vi "current (SubVI).vi"(5 "T_wave":dbl=5.0, 6 "eta in":dbl[](array[numeric]), 7 "zeta_a":dbl, 8 "nu_c_ned in":dbl[](array[numeric])=[0.0, 0.0, 0.0, 0.0, 0.0, 0.0], 9 "dt sim":dbl=10.0, 10 "loop it":i32, 11 "Waves":bool) -> (3 "nu_c_ned out":dbl[](array[numeric]))   [LabVIEW 2014]
uses:
  <vilib>/imath/engines/lvmath2/RunTimeEngine/IndexRead/NIMS V(S).vi
  <instcachedir>/0/NIMS V(S)_0488751826AF41519A22953C041130DC.lvgen/NIMS V(S)_0488751826AF41519A22953C041130DC_000.vi
  <vilib>/imathl/engines/lvmath/Functions/Error Handling/Create Error.vi
  <vilib>/imath/engines/lvmath2/RunTimeEngine/NodeEndStatement/NIMS_NodeEndStatement_Output.vi
  <instcachedir>/0/NIMS_NodeEndStatement_Output_53EC0D466D134D7ABD903AC30B43404B.lvgen/NIMS_NodeEndStatement_Output_53EC0D466D134D7ABD903AC30B43404B_005.vi
  <vilib>/imath/engines/lvmath2/RunTimeEngine/ErrorHandling/NIMS_Finalize Error.vi
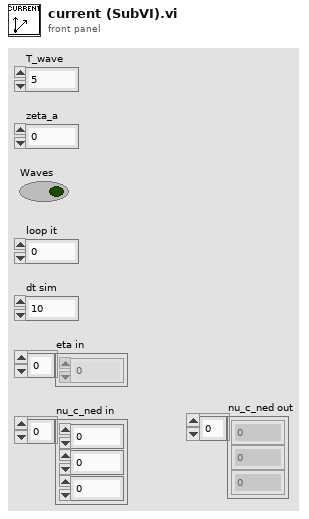
[diagram p1: front panel]
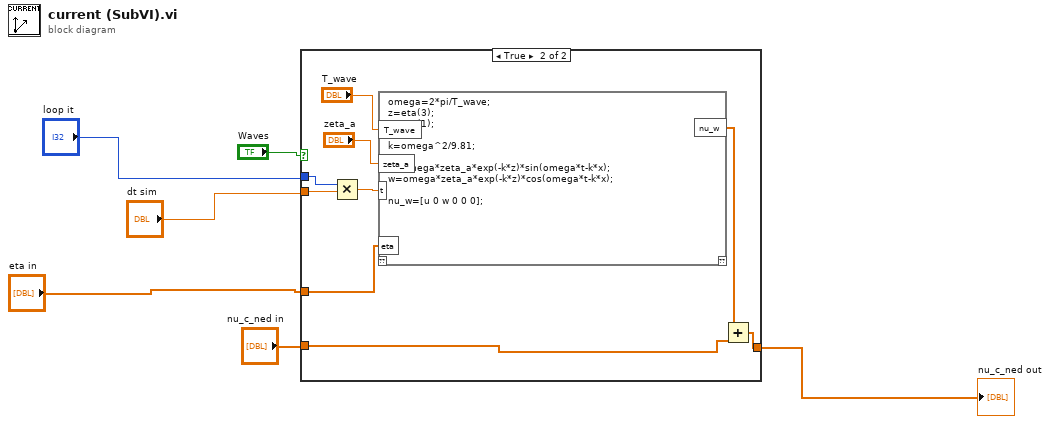
[diagram p0: block diagram]
diagram:
  n1 = case shown="True" "Waves" {
    tunnel: "nu_c_ned in" -> [w7 w10]
    tunnel: [w7 w9] -> w2
    tunnel: "loop it" -> [_ w16]
    tunnel: "dt sim" -> [_ w15]
    tunnel: "eta in" -> [_ w11]
    frame False {
    }
    frame True {
      n2 = Multiply(x=w16, y=w15) -> (x*y=w14:dbl)
      n3 = mathscript code="omega=2*pi/T_wave;\nz=eta(3);\nx=eta(1);\n\nk=omega^2/9.81;\n\nu=omega*zeta_a*exp(-k*z)*sin(omega*t-k*x);\nw=omega*zeta_a*exp(-k*z)*cos(omega*t-k*x);\n\nnu_w=[u 0 w 0 0 0];"("T_wave"="T_wave", "zeta_a"="zeta_a", "t"=w14, "eta"=w11) -> ("nu_w"=w8:dbl[])  [unwired: 1 in, 1 out]
      n4 = Add(x=w8, y=w10) -> (x+y=w9:dbl[])
    }
  }
  "nu_c_ned out" <- w2
